vi "_binary_search.vi"(3 "Indices in (none)":i32[](array[numeric]), 4 "String to search":string, 5 "Strings in":string[](array[string])) -> (1 "Index out":i32)   [LabVIEW 2020, in "Rohde&Schwarz RTx Oscilloscopes.lvlib" / "rsidr_core.lvlib"]
uses:
  rsidr_core.lvlib
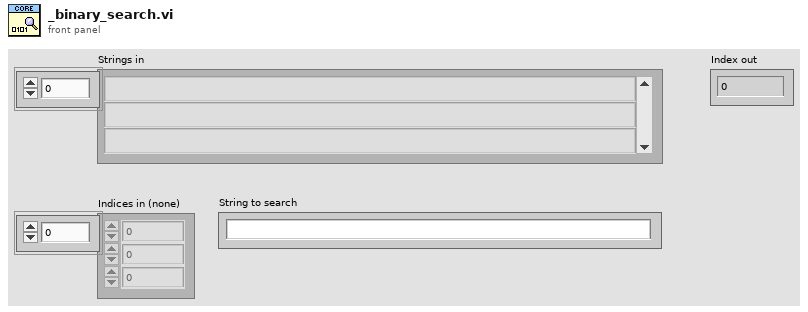
[diagram p1: front panel]
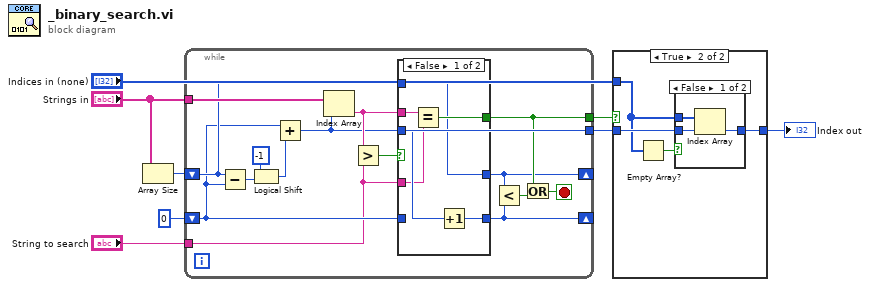
[diagram p0: block diagram]
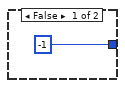
[diagram p2: hidden frame]
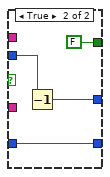
[diagram p4: hidden frame]
diagram:
  n1 = Array Size(array="Strings in") -> (size(s)=w8:i32)
  n2 = while {
    shift-right: [w10] -> _
    shift-left: w8 -> [w19]
    shift-right: [w9] -> _
    shift-left: 0 ("Index") -> [w14]
    tunnel: "String to search" -> [w12]
    tunnel: [w11] -> w5
    tunnel: "Strings in" -> [w23]
    tunnel: [w13] -> w1
    stop <- w22 stop-if-true
    n3 = Subtract(x=w19, y=w14) -> (x-y=w18:i32)
    n4 = Logical Shift(y=-1, x=w18) -> (x << y=w15:i32)
    n5 = Add(x=w14, y=w15) -> (x+y=w13:i32)
    n6 = Index Array(array=w23, index=w13) -> (element=w17:string)
    n7 = Greater?(x=w17, y=w12) -> (0:w20:bool)
    n8 = case shown="False" w20 {
      tunnel: w14 -> [_ w33]
      tunnel: [w26 w33] -> w9
      tunnel: w19 -> [w27 _]
      tunnel: w13 -> [w25 w30]
      tunnel: [w27 w31] -> w10
      tunnel: [w28 FALSE] -> w11
      tunnel: w17 -> [w29 _]
      tunnel: w12 -> [w24 _]
      frame False {
        n9 = Equal?(x=w29, y=w24) -> (x = y?=w28:bool)
        n10 = Increment(x=w25) -> (x+1=w26:i32)
      }
      frame True {
        n11 = Decrement(x=w30) -> (x-1=w31:i32)
      }
    }
    n12 = Less?(x=w10, y=w9) -> (x < y?=w21:bool)
    n13 = Or(x=w11, y=w21) -> (x .or. y?=w22:bool)
  }
  n14 = case shown="True" w5 {
    tunnel: "Indices in (none)" -> [_ w35]
    tunnel: [-1 ("Index") w38] -> w3
    tunnel: w1 -> [_ w36]
    frame False {
    }
    frame True {
      n15 = Empty Array?(array=w35) -> (empty?=w37:bool)
      n16 = case shown="False" w37 {
        tunnel: w35 -> [w41 _]
        tunnel: [w40 w42] -> w38
        tunnel: w36 -> [w39 w42]
        frame False {
          n17 = Index Array(array=w41, index=w39) -> (element=w40:i32)
        }
        frame True {
        }
      }
    }
  }
  "Index out" <- w3
